vi "log execution errors.vi"(8 "error in (no error)":errorcluster, 11 "Channel in":refnum<class "Channel.lvclass">) -> (0 "error out":errorcluster, 3 "Channel out":refnum<class "Channel.lvclass">)   [LabVIEW 2018, in "Channel.lvclass"]
uses:
  Channel.lvclass
  Channel.lvclass/Channel.ctl
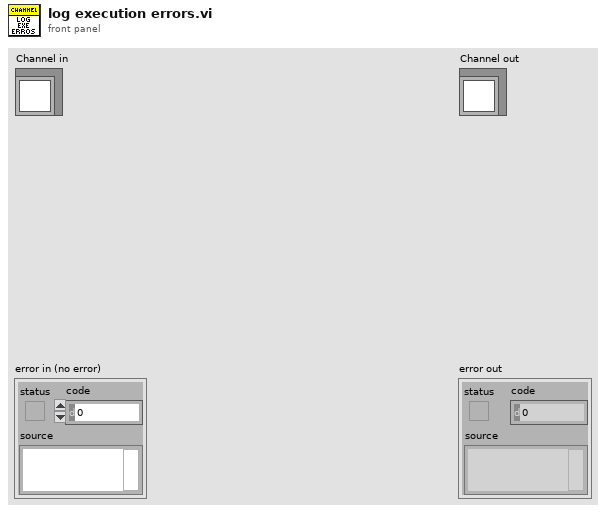
[diagram p1: front panel]
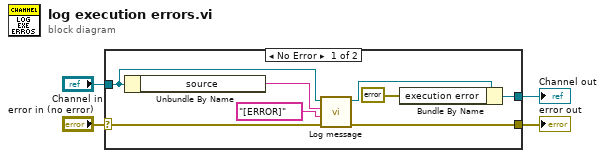
[diagram p0: block diagram]
diagram:
  n1 = case shown="No Error" "error in (no error)" {
    selector: "error in (no error)" -> [w12 w14]
    tunnel: [w10 w14] -> w3
    tunnel: [w6 w13] -> w1
    tunnel: "Channel in" -> [w11 w13]
    frame No Error {
      n2 = Unbundle By Name(w11) -> ("source"=w8:string)
      n3 = call "Log message.vi"("error in (no error)"=w12, "message type"="[ERROR]", "String"=w8, "Channel in"=w11) -> ("error out"=w10:errorcluster, "Channel out"=w7:refnum<class "Channel.lvclass">)  [unwired: 6 in]
      n4 = Bundle By Name(cluster=w7, "execution error"=errorcluster {"status"=FALSE, "code"=0, "source"=""}) -> (w6:refnum<class "Channel.lvclass">)
    }
    frame Error {
    }
  }
  "error out" <- w3
  "Channel out" <- w1
